vi "Straight line from two dots.vi"(8 "Y2":dbl, 9 "X2":dbl, 10 "Y1":dbl, 11 "X1":dbl) -> (0 "X intercept":dbl, 3 "Slope":dbl)   [LabVIEW 2016]
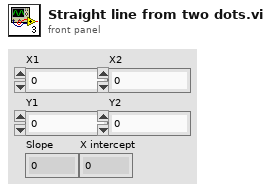
[diagram p1: front panel]
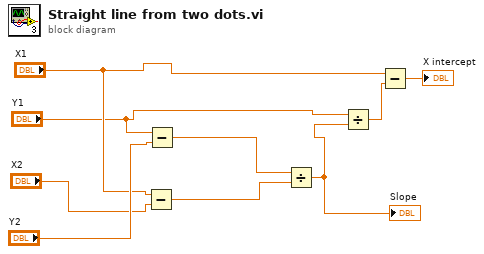
[diagram p0: block diagram]
diagram:
  n1 = Subtract(x="X1", y="X2") -> (x-y=w6:dbl)
  n2 = Subtract(x="Y1", y="Y2") -> (x-y=w7:dbl)
  n3 = Divide(x=w7, y=w6) -> (x/y=w3:dbl)
  "Slope" <- w3
  n4 = Divide(x="Y1", y=w3) -> (x/y=w2:dbl)
  n5 = Subtract(x="X1", y=w2) -> (x-y=→"X intercept":dbl)
